vi "Pane Slider.vi"(0 "User Event in":refnum<user-event>, 5 "Invoke Button":refnum<vi>, 7 "Moving Splitter":refnum<vi>, 9 "Fixed Splitter":refnum<vi>) -> ()   [LabVIEW 2022 SP3, in "TLB` Template.lvlib"]
uses:
  TLB` Template.lvlib
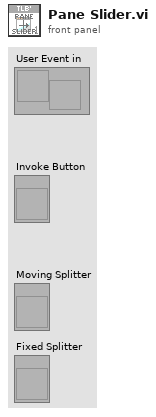
[diagram p1: front panel]
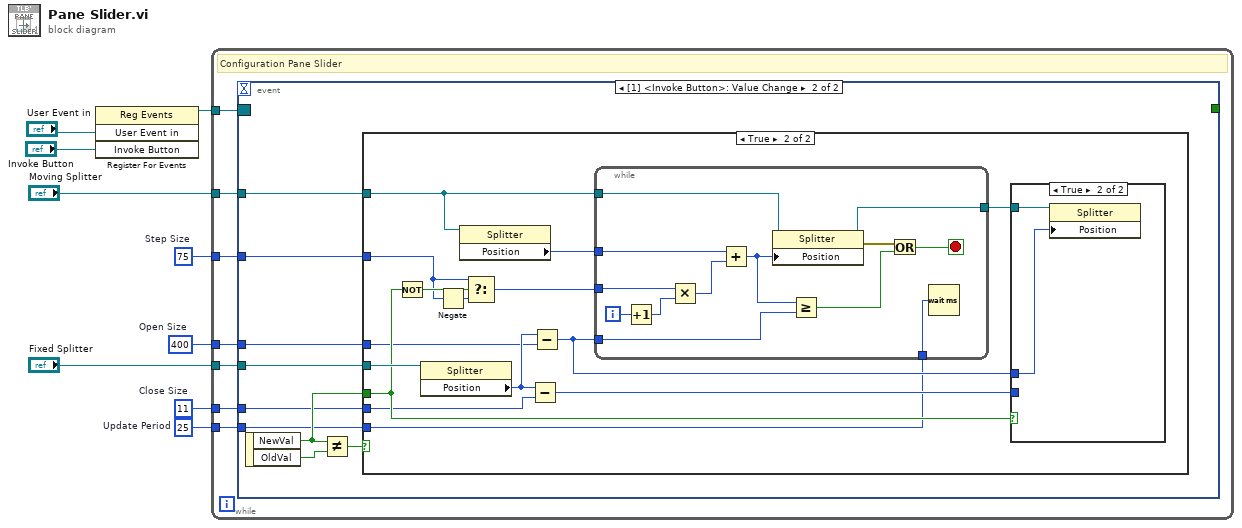
[diagram p0: block diagram]
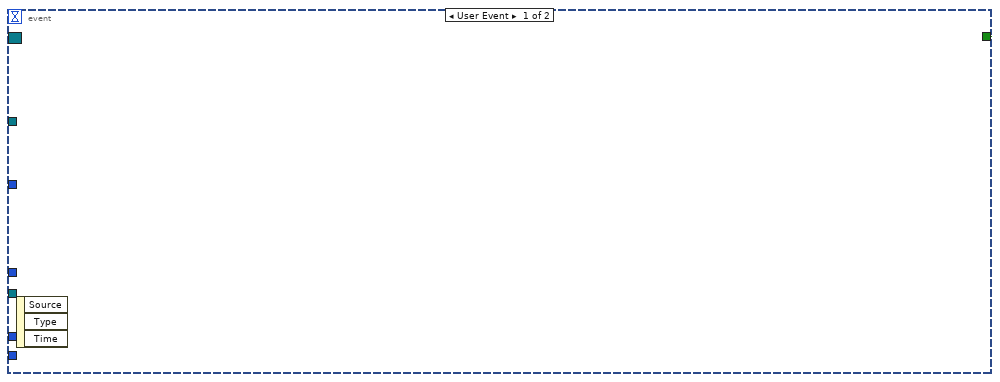
[diagram p2: hidden frame]
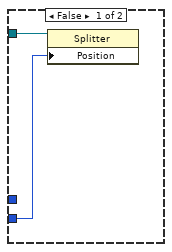
[diagram p4: hidden frame]
diagram:
  w1 = u32 25  # Update Period
  w2 = i16 11  # Close Size
  w3 = i16 400  # Open Size
  w4 = i16 75  # Step Size
  n1 = register-events("User Event in", "Invoke Button") -> (reference out=w7:refnum<event-registration>)  [unwired: 2 in, 1 out]
  n2 = while {
    tunnel: w7 -> [w16]
    tunnel: "Fixed Splitter" -> [w15]
    tunnel: "Moving Splitter" -> [w14]
    tunnel: w4 -> [w13]
    tunnel: w3 -> [w12]
    tunnel: w2 -> [w11]
    tunnel: w1 -> [w10]
    stop <- w17 stop-if-true
    # "Configuration Pane Slider"
    n3 = event shown="[1] <Invoke Button>: Value Change" {
      selector: w16 -> [_ _]
      dyn-events: _ -> [_ _]
      timeout: _ -> [_ _]
      tunnel: [TRUE _] -> w17
      tunnel: w15 -> [_ w24]
      tunnel: w14 -> [_ w23]
      tunnel: w13 -> [_ w22]
      tunnel: w12 -> [_ w21]
      tunnel: w11 -> [_ w20]
      tunnel: w10 -> [_ w19]
      event User Event {
        n4 = event-data() -> ()  [unwired: 1 in, 3 out]
      }
      event Value Change {
        n5 = event-data() -> ("NewVal"=w27:bool, "OldVal"=w25:bool)  [unwired: 1 in]
        n6 = Not Equal?(x=w27, y=w25) -> (x != y?=w26:bool)
        n7 = case shown="True" w26 {
          tunnel: w23 -> [_ w37]
          tunnel: w24 -> [_ w35]
          tunnel: w27 -> [_ w32]
          tunnel: w22 -> [_ w31]
          tunnel: w21 -> [_ w30]
          tunnel: w20 -> [_ w29]
          tunnel: w19 -> [_ w28]
          frame False {
          }
          frame True {
            n8 = Not(x=w32) -> (.not. x?=w36:bool)
            n9 = property class="Splitter"(reference=w35) -> ("Position"=w34:i32)  [unwired: 1 in, 2 out]
            n10 = Negate(x=w31) -> (-x=w38:i16)
            n11 = property class="Splitter"(reference=w37) -> ("Position"=w40:i32)  [unwired: 1 in, 2 out]
            n12 = Select(t=w31, s=w36, f=w38) -> (s? t:f=w39:i16)
            n13 = Subtract(x=w34, y=w29) -> (x-y=w41:i32)
            n14 = Subtract(x=w34, y=w30) -> (x-y=w33:i32)
            n15 = while {
              tunnel: w37 -> [w45]
              tunnel: w39 -> [w54]
              tunnel: w40 -> [w48]
              tunnel: [w44] -> w42
              tunnel: w33 -> [w46]
              tunnel: w28 -> [w43]
              i -> [w55]
              stop <- w52 stop-if-true
              n16 = Increment(x=w55) -> (x+1=w47:i32)
              n17 = Multiply(x=w54, y=w47) -> (x*y=w51:i32)
              n18 = Add(x=w48, y=w51) -> (x+y=w49:i32)
              n19 = property class="Splitter"(reference=w45, "Position"=w49) -> (reference out=w44:refnum<vi>, error out=w53:errorcluster)  [unwired: 1 in]
              n20 = Greater Or Equal?(x=w49, y=w46) -> (x >= y?=w50:bool)
              n21 = Or(x=w53, y=w50) -> (x .or. y?=w52:bool)
              n22 = Wait (ms)(milliseconds to wait=w43) -> ()  [unwired: 1 out]
            }
            n23 = case shown="True" w32 {
              tunnel: w42 -> [w57 w59]
              tunnel: w41 -> [w56 _]
              tunnel: w33 -> [_ w58]
              frame False {
                n24 = property class="Splitter"(reference=w57, "Position"=w56) -> ()  [unwired: 1 in, 2 out]
              }
              frame True {
                n25 = property class="Splitter"(reference=w59, "Position"=w58) -> ()  [unwired: 1 in, 2 out]
              }
            }
          }
        }
      }
    }
  }
